vi "Day 4.1 - .vi"(11 "input":string[](array[string])) -> (3 "output":i16)   [LabVIEW 2021]
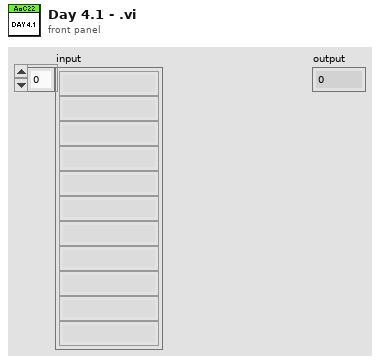
[diagram p1: front panel]
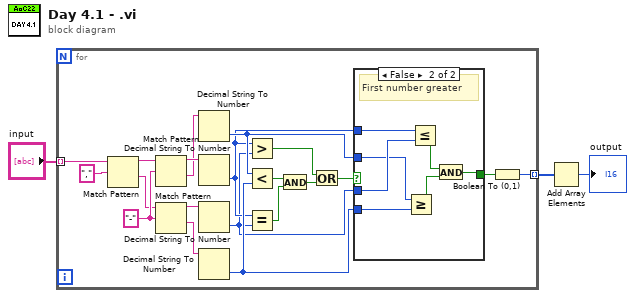
[diagram p0: block diagram]
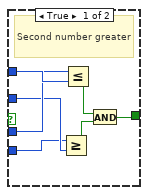
[diagram p2: hidden frame]
diagram:
  n1 = for {
    tunnel: "input" -> [w15] mode=indexing
    tunnel: [w16] -> w2 mode=indexing
    w22 = "-" ("regular expression")
    n2 = Match Pattern(string=w15, regular expression=",") -> (before substring=w14:string, after substring=w13:string)  [unwired: 1 in, 2 out]
    n3 = Match Pattern(string=w14, regular expression=w22) -> (before substring=w21:string, after substring=w20:string)  [unwired: 1 in, 2 out]
    n4 = Match Pattern(string=w13, regular expression=w22) -> (before substring=w19:string, after substring=w18:string)  [unwired: 1 in, 2 out]
    n5 = Decimal String To Number(string=w20) -> (number=w11:i32)  [unwired: 2 in, 1 out]
    n6 = Decimal String To Number(string=w21) -> (number=w9:i32)  [unwired: 2 in, 1 out]
    n7 = Decimal String To Number(string=w19) -> (number=w8:i32)  [unwired: 2 in, 1 out]
    n8 = Decimal String To Number(string=w18) -> (number=w10:i32)  [unwired: 2 in, 1 out]
    n9 = Greater?(x=w9, y=w8) -> (0:w17:bool)
    n10 = Less?(x=w11, y=w10) -> (x < y?=w6:bool)
    n11 = Equal?(x=w9, y=w8) -> (x = y?=w7:bool)
    n12 = And(x=w6, y=w7) -> (x .and. y?=w4:bool)
    n13 = Or(x=w17, y=w4) -> (x .or. y?=w5:bool)
    n14 = case shown="False" w5 {
      tunnel: w9 -> [w30 w37]
      tunnel: w8 -> [w29 w36]
      tunnel: w11 -> [w28 w35]
      tunnel: w10 -> [w27 w34]
      tunnel: [w26 w31] -> w12
      frame True {
        # "Second number greater"
        n15 = Greater Or Equal?(x=w27, y=w28) -> (x >= y?=w24:bool)
        n16 = Less Or Equal?(x=w29, y=w30) -> (x <= y?=w25:bool)
        n17 = And(x=w25, y=w24) -> (x .and. y?=w26:bool)
      }
      frame False {
        # "First number greater"
        n18 = Greater Or Equal?(x=w35, y=w34) -> (x >= y?=w33:bool)
        n19 = Less Or Equal?(x=w37, y=w36) -> (x <= y?=w32:bool)
        n20 = And(x=w32, y=w33) -> (x .and. y?=w31:bool)
      }
    }
    n21 = Boolean To (0,1)(Boolean=w12) -> (0, 1=w16:i16)
  }
  n22 = Add Array Elements(numeric array=w2) -> (sum=→"output":i16)
